vi "TA_Time2Position.vi"(9 "Delay Time (ps)":dbl[](array[numeric])=[0.0, 10.0, 100.0, 1000.0, 2000.0, 3000.0, 4000.0, 5000.0, 6000.0, 7000.0, 8000.0], 10 "Absolute Position of 0 ps (mm)":dbl=50.0, 11 "Number of Optical Path":dbl=2.0) -> (3 "Absolute Position (mm)":dbl[](array[numeric]) format="%.8g")   [LabVIEW 2025]
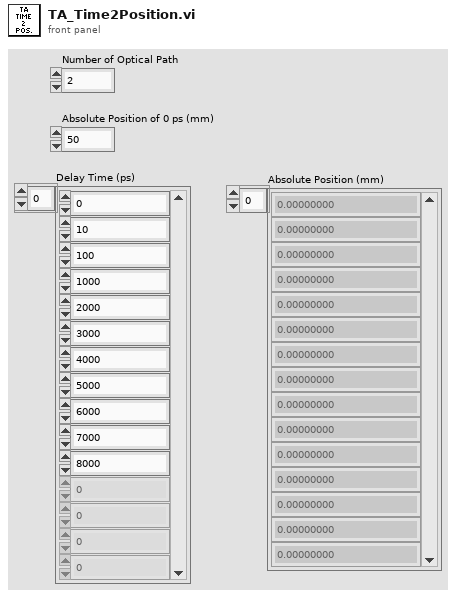
[diagram p1: front panel]
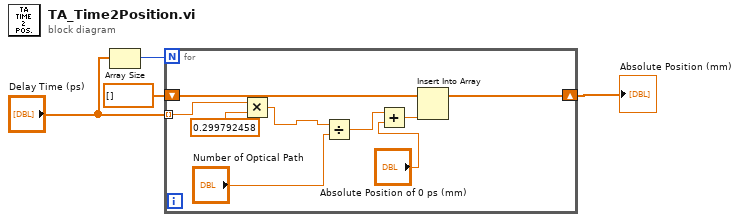
[diagram p0: block diagram]
diagram:
  n1 = Array Size(array="Delay Time (ps)") -> (size(s)=w4:i32)
  n2 = for {
    N: w4 -> [_]
    tunnel: "Delay Time (ps)" -> [w11] mode=indexing
    shift-right: [w12] -> w1
    shift-left: dbl[] [] ("Delay Position (mm)") -> [w13]
    n3 = Multiply(x=w11, y=0.299792458) -> (x*y=w9:dbl)
    n4 = Divide(x=w9, y="Number of Optical Path") -> (x/y=w6:dbl)
    n5 = Add(x=w6, y="Absolute Position of 0 ps (mm)") -> (x+y=w5:dbl)
    n6 = Insert Into Array(array=w13, new element=w5) -> (w12:dbl[])  [unwired: 1 in]
  }
  "Absolute Position (mm)" <- w1
